vi "SeCrTs-AI_Read.vi"(5 "Data FIFO Ref":T1, 6 "error in (no error)":errorcluster, 7 "Numeric":dbl=10.0, 9 "AI_Task":refnum<k21>) -> (0 "error out":errorcluster, 3 "task out":refnum<k21>)   [LabVIEW 2022 SP3]
uses:
  RT Controls/ATF Storage-Data FIFO.ctl
  <vilib>/Platform/TimedLoop/XDataNode/timing_clust.ctl
  <vilib>/Platform/TimedLoop/XDataNode/nitl_modes.ctl
  <vilib>/Platform/TimedLoop/XDataNode/wakeup.ctl
  RT Controls/ATF Storage Haelth.ctl
  <vilib>/DAQmx/read.llb/DAQmx Read (Analog 1D Wfm NChan NSamp).vi
  <vilib>/DAQmx/miscellaneous.llb/DAQmx Fill In Error Info.vi
  <vilib>/platform/TimedLoop/XDataNode/XDataNode.xnode
  <vilib>/Platform/TimedLoop/XDataNode/XDNodeRunTimeDep.lvlib
panel:
  out "x":u32
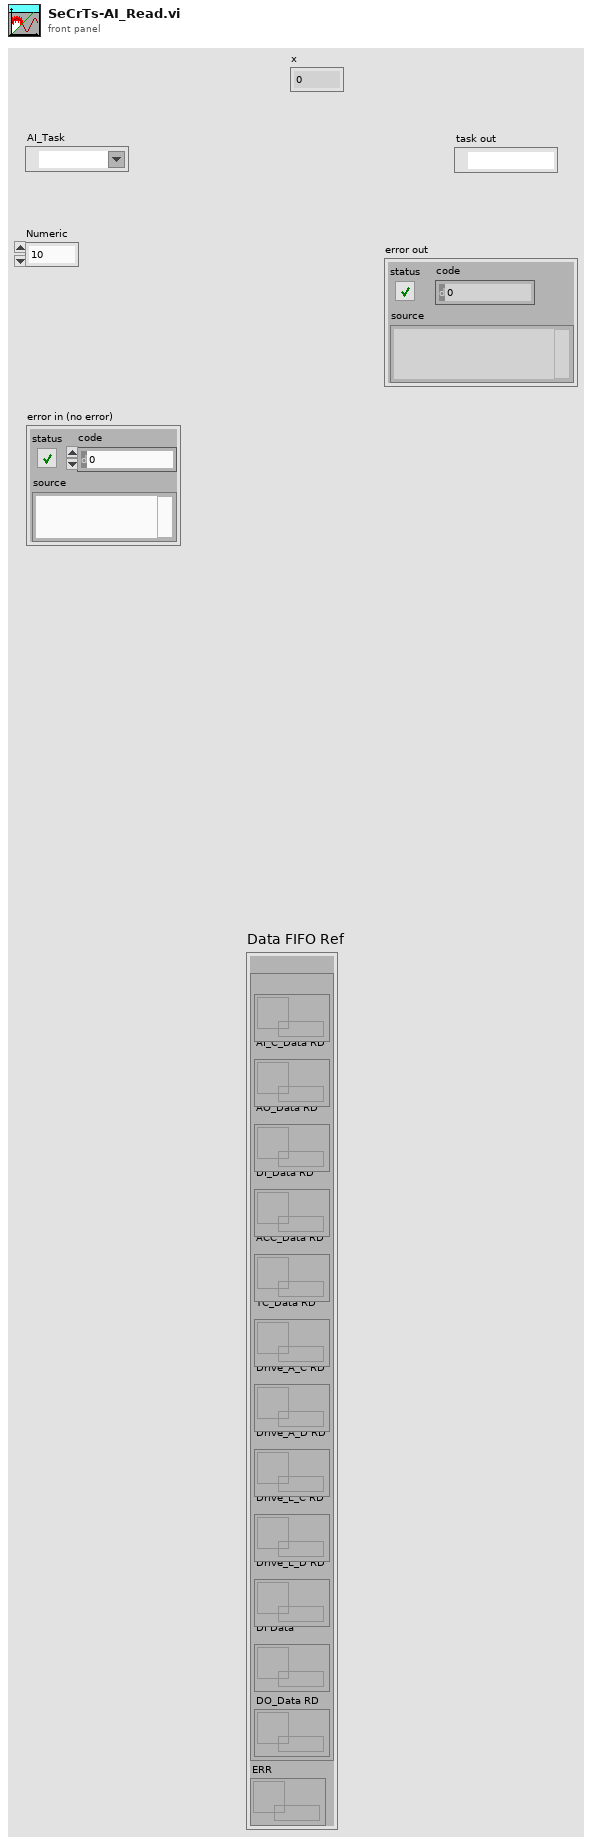
[diagram p1: front panel]
types:
  T1 = typedef "ATF Storage-Data FIFO.ctl" = cluster{"RD":cluster{"AI_V_Data RD":refnum<queue>, "AI_C_Data RD":refnum<queue>, "AO_Data RD":refnum<queue>, "DI_Data RD":refnum<queue>, "ACC_Data RD":refnum<queue>, "TC_Data RD":refnum<queue>, "Drive_A_C RD":refnum<queue>, "Drive_A_D RD":refnum<queue>, "Drive_L_C RD":refnum<queue>, "Drive_L_D RD":refnum<queue>, "DI Data":refnum<queue>, "DO_Data RD":refnum<queue>}, "ERR":refnum<queue>}
  T2 = typedef "XDNodeRunTimeDep.lvlib/timing_clust.ctl" = cluster{"Expected End [f-1]":u64, "Actual End [f-1]":u64, "Finished Late? [f-1]":bool, "Expected End [i-1]":u64, "Actual End [i-1]":u64, "Finished Late? [i-1]":bool, "Expected Start [i]":u64, "Actual Start [i]":u64, "Expected Start [f]":u64, "Actual Start [f]":u64, "Source Name":string, "Structure Name":string, "Period":i64, "Deadline":i64, "Offset":i64, "Start":i64, "Priority":i32, "Timeout":i32, "Mode":T3, "Wakeup Reason":T4, "Error":errorcluster, "Source Type":string, "Secondary Source Type":string, "Global End Time":u64, "Global Start Time":u64, "Frame Duration":u64, "Iteration Duration":u64, "Assigned CPU":i32, "I/O Scan Engine Mode":u32}
  T3 = typedef "XDNodeRunTimeDep.lvlib/nitl_modes.ctl" = enum32{"No Change", "Process missed periods, maintain original phase", "Discard missed periods, maintain original phase", "Process missed periods, ignore original phase", "Discard missed periods, ignore original phase"}
  T4 = typedef "XDNodeRunTimeDep.lvlib/wakeup.ctl" = enum32{"Normal", "Aborted", "Asynchronous wakeup", "Timing source error", "Timed loop error", "Timeout"}
  T5 = typedef "ATF Storage Haelth.ctl" = enum16{"AI C", "AI V", "AO", "DI", "DO", "TC", "ACC", "RT Str", "DR A"}
  T6 = enum16{"Init", "Read 'All'", "Read 'n'", "Read '1'", "Write '1'", "Write 'n'", "Write 'All'"}
  T7 = cluster{"Start DAQ":bool, "Stop DAQ":bool, "RT Stop":bool, "RT Exit":bool, "Start Seq":bool}
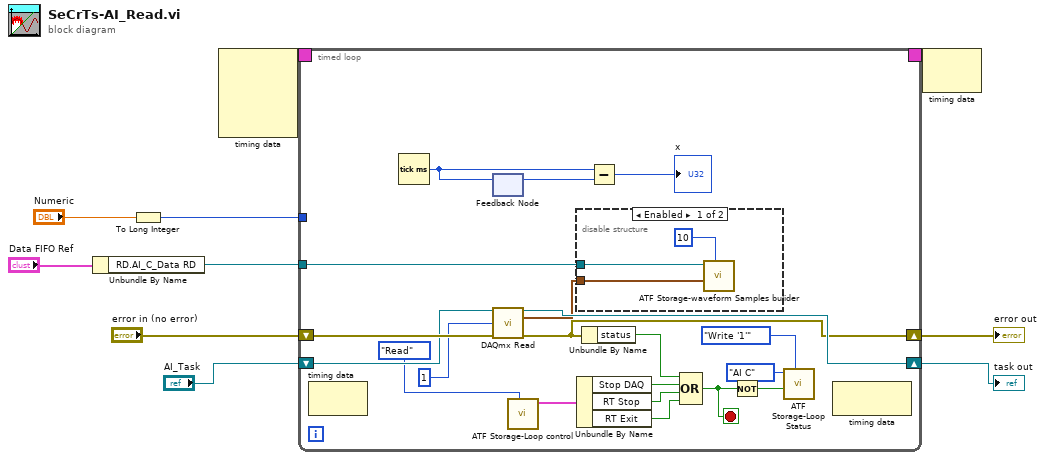
[diagram p0: block diagram]
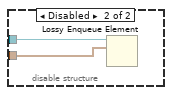
[diagram p2: hidden frame]
diagram:
  n1 = Unbundle By Name("Data FIFO Ref") -> ("RD.AI_C_Data RD"=w3:refnum<queue>)
  n2 = To Long Integer(number="Numeric") -> (32bit integer=w7:i32)
  n3 = node-c288() -> (w2:T2)  [unwired: 4 in]
  n4 = timed-loop {
    tunnel: w7 -> [_]
    shift-right: [w19] -> w6
    shift-left: "AI_Task" -> [w29]
    shift-right: [w16] -> w5
    shift-left: "error in (no error)" -> [w30]
    tunnel: w3 -> [w18]
    timing: w2 -> [_]
    timing-out: [_] -> w1
    stop <- w28 stop-if-true
    n5 = node-c288() -> ()  [unwired: 1 in, 1 out]
    n6 = Tick Count (ms)() -> (millisecond timer value=w15:u32)
    n7 = feedback #1() -> (w14:u32)  [unwired: 1 in]
    n8 = feedback-in #1(w15) -> ()
    n9 = call-poly <vilib>:"DAQmx Read.vi"("task/channels in"=w29, "number of samples per channel"=1, "error in"=w30) -> ("task out"=w19:refnum<k21>, "data"=w17:waveform(dbl)[], "error out"=w16:errorcluster)  [unwired: 10 in]
    n10 = call "ATF Storage-Loop control.vi"("Action"=enum16{"Init", "Write", "Read"}."Read") -> ("Loop Control out"=w26:T7)  [unwired: 9 in, 1 out]
    n11 = disable-structure shown="Enabled" {
      disable-tunnel: w18 -> [w35 w37]
      disable-tunnel: w17 -> [w33 w36]
      frame Enabled {
        n12 = call "ATF Storage-waveform Samples bulider.vi"("Samples"=10, "Data input"=w33, "AI_C_Data RD"=w35) -> ()  [unwired: 8 in, 1 out]
      }
      frame Disabled {
        n13 = Lossy Enqueue Element(queue=w37, element=w36) -> ()  [unwired: 1 in, 4 out]
      }
    }
    n14 = Unbundle By Name(w26) -> ("Stop DAQ"=w25:bool, "RT Stop"=w24:bool, "RT Exit"=w23:bool)
    n15 = Unbundle By Name(w16) -> ("status"=w27:bool)
    n16 = Subtract(x=w15, y=w14) -> (x-y=→"x":u32)
    n17 = Compound Arithmetic op=OR(w27, w25, w24, w23) -> (w28:bool)
    n18 = Not(x=w28) -> (.not. x?=w20:bool)
    n19 = call "ATF Storage-Loop Status.vi"("Option"=T6."Write '1'", "Status"=w20, "Loop"=ATF_Storage_Haelth."AI C") -> ()  [unwired: 6 in, 3 out]
    n20 = node-c288() -> ()  [unwired: 1 in, 1 out]
  }
  "task out" <- w6
  "error out" <- w5
  n21 = node-c288(w1) -> ()  [unwired: 1 out]
